vi "Is Sleeping.vi"(8 "error in (no error)":errorcluster, 11 "ISleepableBaby in":refnum<class "ISleepableBaby.lvclass">) -> (0 "error out":errorcluster, 2 "IsSleeping":bool, 3 "ISleepableBaby out":refnum<class "ISleepableBaby.lvclass">)   [LabVIEW 2009, in "ISleepableBaby.lvclass"]
doc: "Check on baby to see if she's sleeping."
uses:
  ISleepableBaby.lvclass
  Baby.lvclass
  Source/IUnknown Class/IUnknown.lvclass
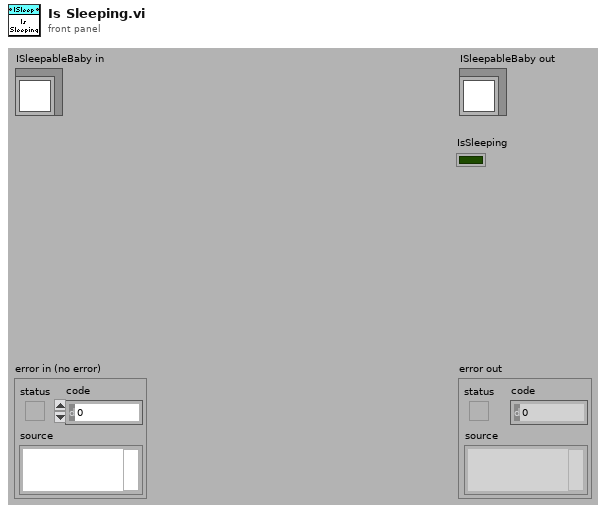
[diagram p1: front panel]
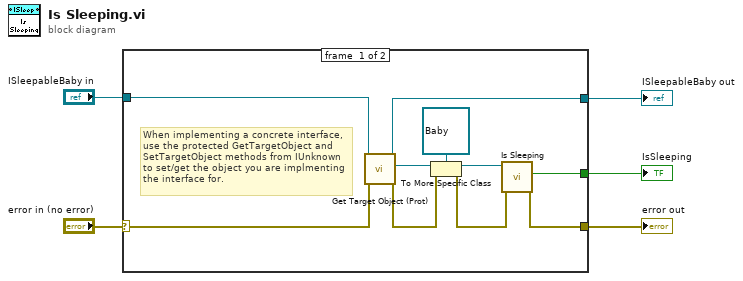
[diagram p0: block diagram]
diagram:
  n1 = case shown="No Error" "error in (no error)" {
    selector: "error in (no error)" -> [w9 w17]
    tunnel: "ISleepableBaby in" -> [w15 w16]
    tunnel: [w14 _] -> w4
    tunnel: [w13 w16] -> w3
    tunnel: [w6 w17] -> w2
    frame #0 {
      # "When implementing a concrete interface,\nuse the protected GetTargetObject and SetTargetObject methods from IUnknown to set/get the object you are implmenting the interface for."
      n2 = call "Get Target Object (Prot).vi"("error in (no error)"=w9, "IUnknown in"=w15) -> ("error out"=w8:errorcluster, "Target Object"=w10:refnum<class "Interfaceable.lvclass">, "IUnknown out"=w13:refnum<class "ISleepableBaby.lvclass">)  [unwired: 7 in]
      n3 = To More Specific Class(target class=refnum<class "Baby.lvclass"> refnum ("Baby"), reference=w10, error in=w8) -> (specific class reference=w11:refnum<class "Baby.lvclass">, error out=w7:errorcluster)
      n4 = call "Is Sleeping.vi"("error in (no error)"=w7, "Baby in"=w11) -> ("error out"=w6:errorcluster, "IsSleeping"=w14:bool)  [unwired: 7 in, 1 out]
    }
    frame #1 {
    }
  }
  "error out" <- w2
  "ISleepableBaby out" <- w3
  "IsSleeping" <- w4
